vi "Format String Control.vi"(6 "Format String":string, 8 "error in":errorcluster, 11 "GObject in":refnum<vi>) -> (0 "error out":errorcluster, 2 "Successful":bool)   [LabVIEW 2019, in "Quick Format QD.lvlib"]
doc: "Formats a string control based on the given Format String."
uses:
  Quick Format QD.lvlib
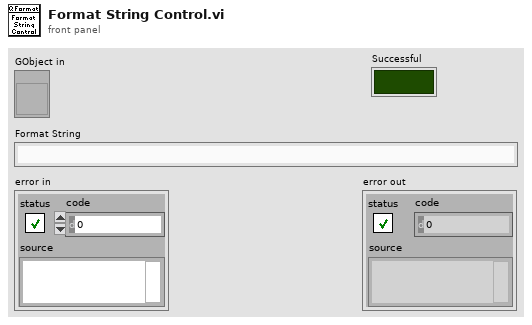
[diagram p1: front panel]
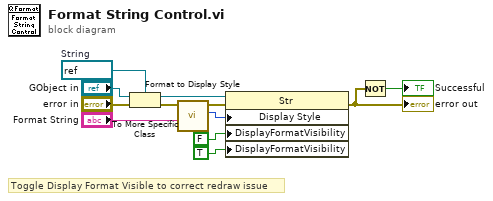
[diagram p0: block diagram]
diagram:
  w8 = refnum<vi> refnum  # String
  # "Toggle Display Format Visible to correct redraw issue"
  n1 = To More Specific Class(target class=w8, reference="GObject in", error in="error in") -> (specific class reference=w5:refnum<vi>, error out=w10:errorcluster)
  n2 = call "Format to Display Style.vi"("Format String"="Format String", "error in"=w10) -> ("Display Style"=w4:u32, "error out"=w9:errorcluster)  [unwired: 8 in]
  n3 = property on="Property Node" class="Str"(reference=w5, error in=w9, "Display Style"=w4, "DisplayFormatVisibility"=FALSE ("Display Format Visible?"), "DisplayFormatVisibility"=TRUE ("Display Format Visible?")) -> (error out=w11:errorcluster)  [unwired: 1 out]
  "error out" <- w11
  n4 = Not(x=w11) -> (.not. x?=→"Successful":bool)
